vi "流程文件XML解析.vi"(5 "简易流程Id":u16(ring), 7 "是否是简易流程":bool, 10 "添加的路径":path, 11 "参数簇":T2={"启动参数"=1, "启动模式"=enum."跨度核查", "量程"=enum."低量程"} {"启动参数" items=["总磷"=1, "总氮"=2, "氨氮"=3]}) -> (2 "通讯数据":u16[](array[numeric]) format="%04xH", 3 "数组":T1(array[cluster]) {"port" format="%08x"})   [LabVIEW 2016, in "斯坦道总磷总氮V2.lvlib"]
uses:
  <vilib>/xml/Load XML File.vi
  <vilib>/xml/Close Reference(Node).vi
  D:/Program Files (x86)/National Instruments/LabVIEW 2016/resource/objmgr/DOMUserDefRef.rc
  <vilib>/xml/NI_XML.lvlib
panel:
  out "字符串":string
  out "大小":i32
  out "XML字符串":string="<?xml version=\"1.0\" encoding=\"ISO-8859-1\"?>\n<bookstore>\n<book ISBN=\"978-0545128285\">\n  <title lang=\"en\">The Tales of Beedle the Bard</title>\n  <author>J. K. Rowling</author>\n  <year>2008</year>\n  <price>12.99</price>\n</book>\n<book ISBN=\"978-0316160209\">\n  <title lang=\"en\">Eclipse</title>\n  <author>Stephenie Meyer</author>\n  <year>2007</year>\n  <price>19.99</price>\n</book>\n<book ISBN=\"978-0316067928\">\n  <title lang=\"en\">Breaking Dawn</title>\n  <author>Stephenie Meyer</author>\n  <year>2008</year>\n  <price>22.99</price>\n</book>\n<book ISBN=\"978-0316017923\">\n  <title lang=\"en\">Outliers: The Story of Success</title>\n  <author>Malcolm Gladwell</author>\n  <year>2008</year>\n  <price>27.99</price>\n</book>\n<book ISBN=\"978-0596007645\">\n  <title lang=\"en\">XML in a Nutshell</title>\n  <author>Elliotte Rusty Harold</author>\n  <author>W. Scott Means</author>\n  <year>2004</year>\n  <price>39.95</price>\n</book>\n</bookstore>"
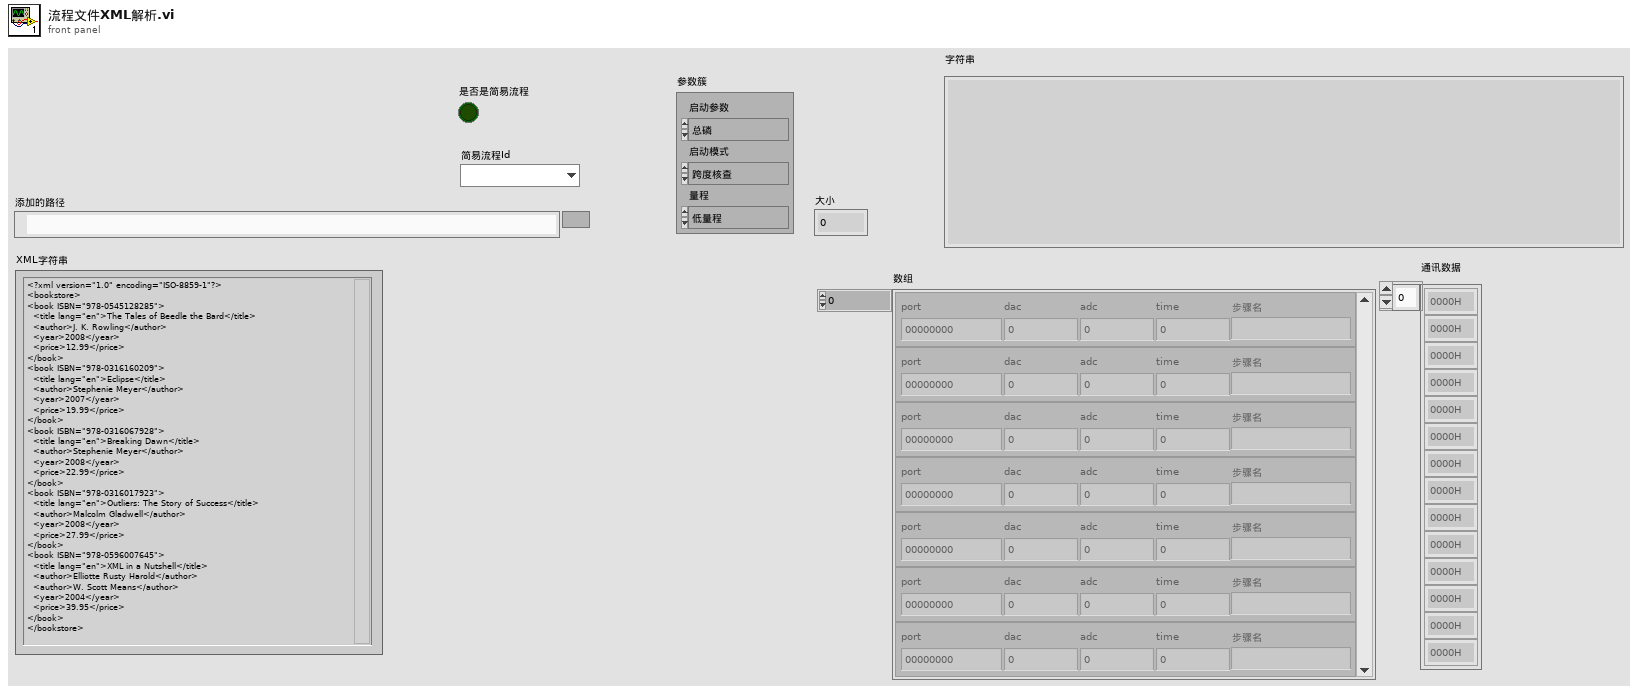
[diagram p1: front panel]
types:
  T1 = cluster{"port":i32, "dac":u8, "adc":u8, "time":u16, "步骤名":string}[]
  T2 = cluster{"启动参数":u16, "启动模式":enum16{"跨度核查", "水样测量", "零点核查", "标样核查", "加标回收", "快捷测试", "空白校准", "标样校准"}, "量程":enum16{"低量程", "高量程"}}
  T3 = cluster{"port":i32, "dac":u8, "adc":u8, "time":u16, "步骤名":string}
  T4 = enum16{"跨度核查", "水样测量", "零点核查", "标样核查", "加标回收", "快捷测试", "空白校准", "标样校准"}
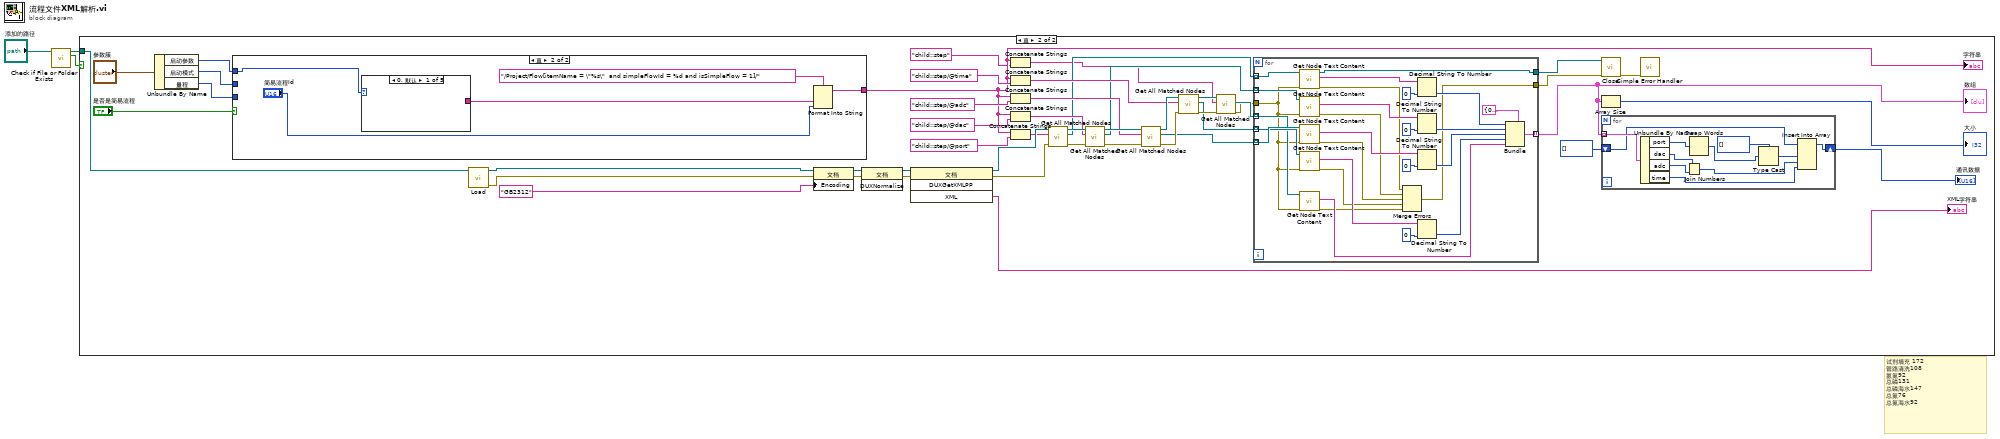
[diagram p0: block diagram]
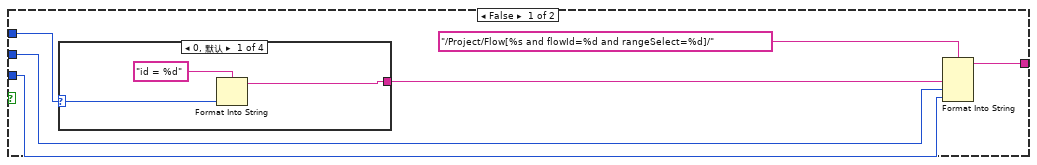
[diagram p3: hidden frame]
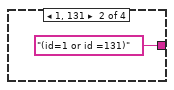
[diagram p4: hidden frame]
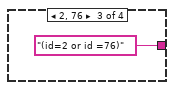
[diagram p5: hidden frame]
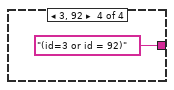
[diagram p6: hidden frame]
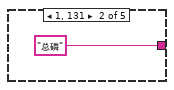
[diagram p7: hidden frame]
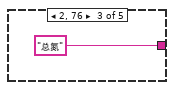
[diagram p8: hidden frame]
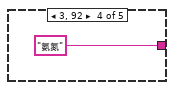
[diagram p9: hidden frame]
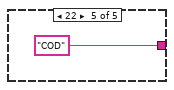
[diagram p10: hidden frame]
diagram:
  # "试剂填充 172 \n管路清洗108\n氨氮92\n总磷131\n总磷海水147\n总氮76\n总氮海水92"
  n1 = call <vilib>:"Check if File or Folder Exists.vi"("path"="添加的路径") -> ("file or folder exists?"=w1:bool, "dup path"=w2:path)  [unwired: 8 in, 1 out]
  n2 = case shown="真" w1 {
    tunnel: w2 -> [_ w37]
    frame False {
    }
    frame True {
      n3 = Unbundle By Name("参数簇") -> ("启动参数"=w38:u16, "启动模式"=w41:T4, "量程"=w40:enum16{"低量程", "高量程"})
      n4 = case shown="真" "是否是简易流程" {
        tunnel: w41 -> [w67 _]
        tunnel: w40 -> [w66 _]
        tunnel: w38 -> [w65 w78]
        tunnel: [w63 w76] -> w19
        frame False {
          n5 = case shown="0, 默认" w65 {
            selector: w65 -> [w70 _ _ _]
            tunnel: [w69 "(id=1 or id =131)" ("输入 4") "(id=2 or id =76)" ("输入 4") "(id=3 or id = 92)" ("输入 4")] -> w64
            frame 0, Default {
              n6 = Format Into String(format string="id = %d" ("格式字符串"), w70) -> (resulting string=w69:string)  [unwired: 2 in, 1 out]
            }
            frame 1, 131 {
            }
            frame 2, 76 {
            }
            frame 3, 92 {
            }
          }
          n7 = Format Into String(format string="/Project/Flow[%s and flowId=%d and rangeSelect=%d]/" ("XPath expression"), w64, w67, w66) -> (resulting string=w63:string)  [unwired: 2 in, 1 out]
        }
        frame True {
          n8 = case shown="0, 默认" w78 {
            tunnel: [_ "总磷" ("输入 4") "总氮" ("输入 4") "氨氮" ("输入 4") "COD" ("输入 4")] -> w77
            frame 0, Default {
            }
            frame 1, 131 {
            }
            frame 2, 76 {
            }
            frame 3, 92 {
            }
            frame 22 {
            }
          }
          n9 = Format Into String(format string="/Project/Flow[itemName = \"%s\"  and simpleFlowId = %d and isSimpleFlow = 1]/" ("XPath expression"), w77, "简易流程Id") -> (resulting string=w76:string)  [unwired: 2 in, 1 out]
        }
      }
      "字符串" <- w19
      n10 = call-poly <vilib>:"Load.vi"("path to XML document"=w37) -> ("DOM document out"=w49:refnum<k20>, "error out"=w48:errorcluster)  [unwired: 12 in, 1 out]
      n11 = property on="属性节点" class="文档"(reference=w49, error in=w48, "Encoding"="GB2312" ("文档编码")) -> (reference out=w47:refnum<k20>, error out=w46:errorcluster)
      n12 = invoke on="Invoke Node" class="文档" method="DUXNormalize"(reference=w47, error in=w46) -> (reference out=w44:refnum<k20>, error out=w45:errorcluster)  [unwired: 1 in, 1 out]
      n13 = invoke on="Invoke Node" class="文档" method="DUXGetXMLPP"(reference=w44, error in=w45) -> (reference out=w36:refnum<k20>, error out=w10:errorcluster, "XML"=→"XML字符串":string)  [unwired: 2 in, 1 out]
      n14 = Concatenate Strings(w19, "child::step" ("输入 4")) -> (w12:string)
      n15 = Concatenate Strings(w19, "child::step/@time" ("输入 4")) -> (w21:string)
      n16 = Concatenate Strings(w19, "child::step/@adc" ("输入 4")) -> (w23:string)
      n17 = Concatenate Strings(w19, "child::step/@dac" ("输入 4")) -> (w25:string)
      n18 = Concatenate Strings(w19, "child::step/@port" ("输入 4")) -> (w35:string)
      n19 = call <vilib>:"Get All Matched Nodes.vi"("error in (no error)"=w10, "XPath expression"=w35, "node in"=w36) -> ("error out"=w32:errorcluster, "node result array"=w17:refnum<k20>[], "node out"=w33:refnum<k20>)  [unwired: 6 in]
      n20 = call <vilib>:"Get All Matched Nodes.vi"("error in (no error)"=w32, "XPath expression"=w25, "node in"=w33) -> ("error out"=w31:errorcluster, "node result array"=w16:refnum<k20>[], "node out"=w30:refnum<k20>)  [unwired: 6 in]
      n21 = call <vilib>:"Get All Matched Nodes.vi"("error in (no error)"=w31, "XPath expression"=w23, "node in"=w30) -> ("error out"=w29:errorcluster, "node result array"=w15:refnum<k20>[], "node out"=w28:refnum<k20>)  [unwired: 6 in]
      n22 = call <vilib>:"Get All Matched Nodes.vi"("error in (no error)"=w29, "XPath expression"=w21, "node in"=w28) -> ("error out"=w27:errorcluster, "node result array"=w14:refnum<k20>[], "node out"=w26:refnum<k20>)  [unwired: 6 in]
      n23 = call <vilib>:"Get All Matched Nodes.vi"("error in (no error)"=w27, "XPath expression"=w12, "node in"=w26) -> ("error out"=w11:errorcluster, "node result array"=w13:refnum<k20>[])  [unwired: 6 in, 1 out]
      n24 = for {
        tunnel: w17 -> [w111] mode=indexing
        tunnel: w16 -> [w110] mode=indexing
        tunnel: w15 -> [w109] mode=indexing
        tunnel: w14 -> [w108] mode=indexing
        tunnel: w13 -> [w107] mode=indexing
        tunnel: [w93] -> w5 mode=indexing
        tunnel: w11 -> [w87]
        tunnel: [w86] -> w9
        tunnel: [w85] -> w8
        n25 = call <vilib>:"Get Node Text Content.vi"("error in (no error)"=w87, "node in"=w111) -> ("error out"=w92:errorcluster, "node text"=w106:string, "node out"=w85:refnum<k20>)  [unwired: 7 in]
        n26 = call <vilib>:"Get Node Text Content.vi"("error in (no error)"=w87, "node in"=w110) -> ("error out"=w91:errorcluster, "node text"=w103:string)  [unwired: 7 in, 1 out]
        n27 = call <vilib>:"Get Node Text Content.vi"("error in (no error)"=w87, "node in"=w109) -> ("error out"=w90:errorcluster, "node text"=w100:string)  [unwired: 7 in, 1 out]
        n28 = call <vilib>:"Get Node Text Content.vi"("error in (no error)"=w87, "node in"=w108) -> ("error out"=w89:errorcluster, "node text"=w99:string)  [unwired: 7 in, 1 out]
        n29 = call <vilib>:"Get Node Text Content.vi"("error in (no error)"=w87, "node in"=w107) -> ("error out"=w88:errorcluster, "node text"=w94:string)  [unwired: 7 in, 1 out]
        n30 = Merge Errors(w92, w91, w90, w89, w88) -> (w86:errorcluster)
        n31 = Decimal String To Number(string=w106, default (0L)=0 ("默认(0 I32)")) -> (number=w98:i32)  [unwired: 1 in, 1 out]
        n32 = Decimal String To Number(string=w103, default (0L)=u8 0 ("默认(0 I32)")) -> (number=w97:u8)  [unwired: 1 in, 1 out]
        n33 = Decimal String To Number(string=w100, default (0L)=u8 0 ("默认(0 I32)")) -> (number=w96:u8)  [unwired: 1 in, 1 out]
        n34 = Decimal String To Number(string=w99, default (0L)=u16 0 ("默认(0 I32)")) -> (number=w95:u16)  [unwired: 1 in, 1 out]
        n35 = Bundle(cluster=T3 {"port"=0, "dac"=0, "adc"=0, "time"=0, "步骤名"=""} ("簇 2"), "port"=w98, "dac"=w97, "adc"=w96, "time"=w95, "步骤名"=w94) -> (w93:T3)
      }
      "数组" <- w5
      n36 = call-poly <vilib>:"Close.vi"("error in (no error)"=w9, "node"=w8) -> ("error out"=w43:errorcluster)  [unwired: 7 out]
      n37 = Array Size(array=w5) -> (size(s)=→"大小":i32)
      n38 = for {
        tunnel: w5 -> [w62] mode=indexing
        shift-right: [w57] -> w4
        shift-left: u16[] [] -> [w55]
        n39 = Unbundle By Name(w62) -> ("port"=w60:i32, "dac"=w52:u8, "adc"=w53:u8, "time"=w58:u16)
        n40 = Join Numbers(hi=w52, lo=w53) -> ((hi.lo)=w59:u16)
        n41 = Swap Words(1:w60) -> (0:w54:i32)
        n42 = Type Cast(type=u16[] [], x=w54) -> (*(type *) &x=w56:u16[])
        n43 = Insert Into Array(array=w55, new element #1=w56, new element #2=w59, new element #3=w58) -> (w57:u16[])  [unwired: 1 in]
      }
      "通讯数据" <- w4
      n44 = call <vilib>:"Simple Error Handler.vi"("error in (no error)"=w43) -> ()  [unwired: 4 in, 5 out]
    }
  }
